vi "SVL Power in Band.vi"   [LabVIEW 2017]
doc: "Computes the aggregate power in the <B>range</B>. The SVL Power in Band VI operates on Power, PSD, COP, and FFT [Mag] spectra. You can use this polymorphic VI to analyze a single spectrum or N spectra. The data type you wire to the <B>spectrum</B> input determines the polymorphic instance to use."
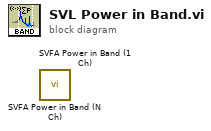
[diagram p0: block diagram]
diagram:
  n1 = call <vilib>:"SVFA Power in Band (N Ch).vi"() -> ()  [unwired: 17 in, 3 out]
  n2 = call <vilib>:"SVFA Power in Band (1 Ch).vi"() -> ()  [unwired: 17 in, 3 out]
